vi "Load and Save Data (FSK Data).vi"(0 "VISA resource name":refnum<visa-resource-name>, 2 "Differential States Count (2)":u32=2, 5 "Destination File":string, 7 "Frequency States Count (2)":u32=2, 9 "Frequency States (Hz)":dbl[](array[numeric])=[0.0, 0.0], 11 "error in (no error)":errorcluster, 12 "Enable Differential Encoding (F:Disable)":bool, 13 "Differential States":dbl[](array[numeric])=[0.0, 0.0]) -> (4 "VISA resource name out":refnum<visa-resource-name>, 15 "error out":errorcluster)   [LabVIEW 2018, in "Agilent PSG MXG Series.lvlib"]
doc: "Loads custom frequency shift keying (FSK) data into a file in the signal generator's non-volatile memory.\n\n<B>Notes:</B>\n(1) This VI is valid in N5172B that installs with <B>Option 653</B> or <B>Option 655</B>, or N5182B that installs with <B>Option 656</B> or <B>Option 657</B>.\n(2) This VI is valid in N5162A/82A that installs with <B>Option 651</B>, <B>Option 652</B>, or <B>Option 654</B>."
uses:
  Agilent PSG MXG Series.lvlib
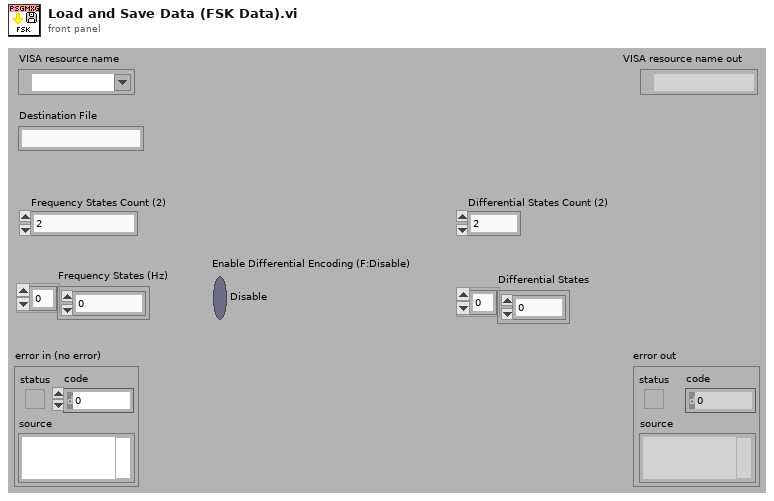
[diagram p1: front panel]
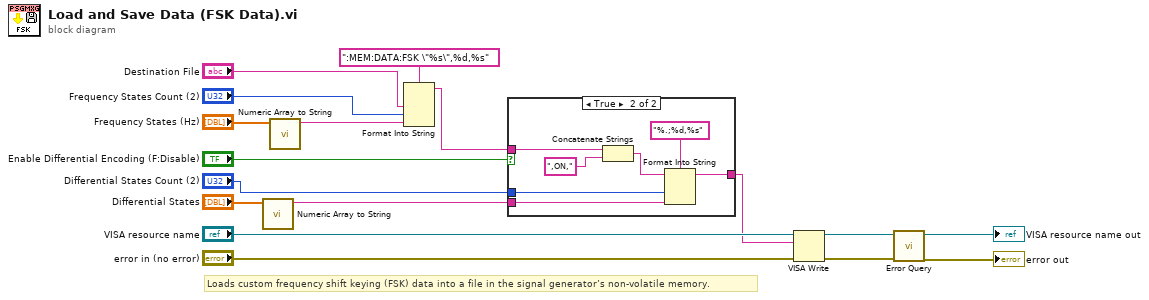
[diagram p0: block diagram]
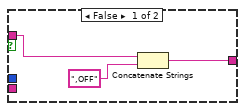
[diagram p2: hidden frame]
diagram:
  # "Loads custom frequency shift keying (FSK) data into a file in the signal generator’s non-volatile memory."
  n1 = call "Numeric Array to String.vi"("Numeric Array"="Differential States") -> ("Output String"=w2:string)  [unwired: 10 in]
  n2 = call "Numeric Array to String.vi"("Numeric Array"="Frequency States (Hz)") -> ("Output String"=w7:string)  [unwired: 10 in]
  n3 = Format Into String(format string=":MEM:DATA:FSK \"%s\",%d,%s", "Destination File", "Frequency States Count (2)", w7) -> (resulting string=w4:string)  [unwired: 2 in, 1 out]
  n4 = case shown="True" "Enable Differential Encoding (F:Disable)" {
    tunnel: w4 -> [w20 w26]
    tunnel: [w18 w21] -> w3
    tunnel: w2 -> [_ w22]
    tunnel: "Differential States Count (2)" -> [_ w23]
    frame False {
      n5 = Concatenate Strings(w20, ",OFF" ("f")) -> (w18:string)
    }
    frame True {
      n6 = Concatenate Strings(w26, ",ON,") -> (w25:string)
      n7 = Format Into String(format string="%.;%d,%s", initial string=w25, w23, w22) -> (resulting string=w21:string)  [unwired: 1 in, 1 out]
    }
  }
  n8 = VISA Write(VISA resource name="VISA resource name", write buffer=w3, error in (no error)="error in (no error)") -> (VISA resource name out=w17:refnum<visa-resource-name>, error out=w16:errorcluster)  [unwired: 1 out]
  n9 = call "Error Query.vi"("error in (no error)"=w16, "VISA resource name"=w17) -> ("error out"=→"error out":errorcluster, "VISA resource name out"=→"VISA resource name out":refnum<visa-resource-name>)  [unwired: 6 in, 2 out]
